vi "Material-ConfigPage-SendMessageToDisplay.vi"(0 "Configuration Page":refnum<class "Material-ConfigPage.lvclass">, 5 "Message to Display":string, 11 "error in":errorcluster) -> (4 "Configuration Page out":refnum<class "Material-ConfigPage.lvclass">, 15 "error out":errorcluster)   [LabVIEW 2013, in "Material-ConfigPage.lvclass"]
uses:
  Material-ConfigPage.lvclass
panel:
  # "Inputs"
  # "Outputs"
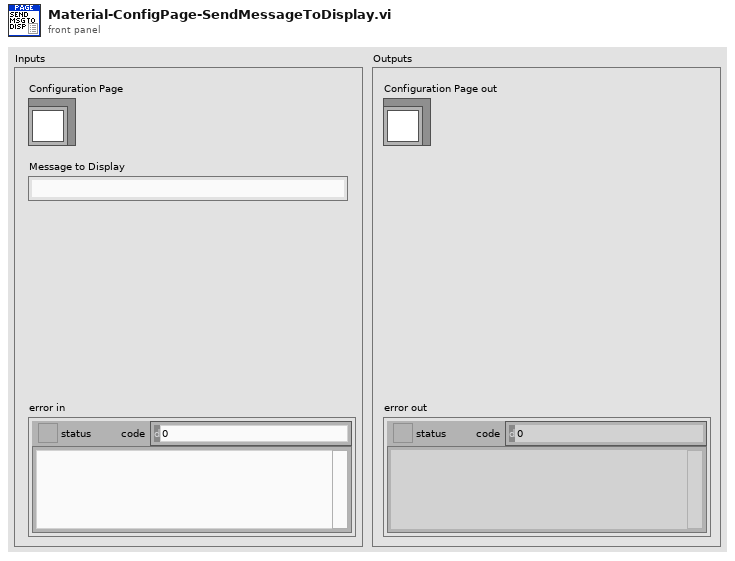
[diagram p1: front panel]
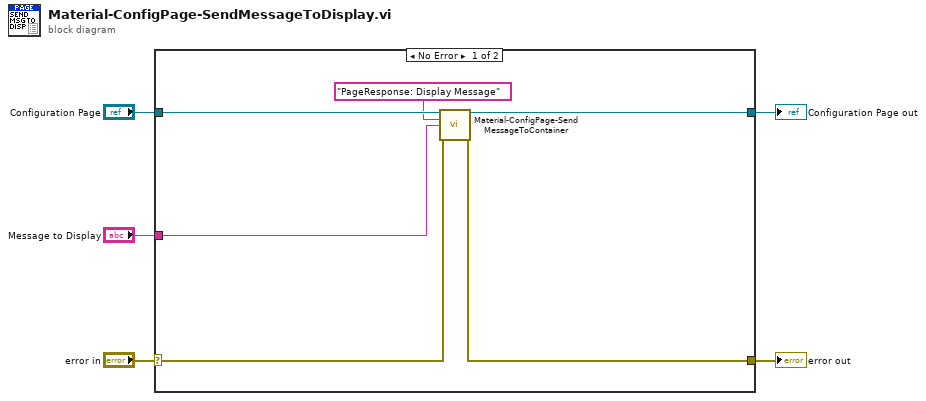
[diagram p0: block diagram]
diagram:
  n1 = case shown="No Error" "error in" {
    selector: "error in" -> [w10 w13]
    tunnel: [w8 w13] -> w5
    tunnel: [w9 w12] -> w3
    tunnel: "Configuration Page" -> [w11 w12]
    tunnel: "Message to Display" -> [w7 _]
    frame No Error {
      n2 = call "Material-ConfigPage-SendMessageToContainer.vi"("Configuration Page"=w11, "Parameter"="PageResponse: Display Message", "Payload"=w7, "error in"=w10) -> ("Configuration Page out"=w9:refnum<class "Material-ConfigPage.lvclass">, "error out"=w8:errorcluster)  [unwired: 10 in]
    }
    frame Error {
    }
  }
  "error out" <- w5
  "Configuration Page out" <- w3
